vi "Image_Capture.vi"() -> ()   [LabVIEW 2017]
uses:
  <vilib>/vision/NI_Vision_Development_Module.lvlib
panel:
  out "error out":errorcluster
  out "Histogram Report":T1 {"Standard  Variation" format="%.2f"; "Mean Value" format="%.2f"; "Interval Width" format="%.2f"; "Starting Value" format="%.2f"; "Maximal Value" format="%.2f"; "Minimal Value" format="%.2f"}
  in  "Contrast::Value":dbl min=0.0 max=1.0
  in  "Brightness::Value":i64=116 min=0 max=255 step=1
  out "Frame Rate":dbl
  in  "Stop (F)":bool
  out "Image Out":T2(plugin-control)
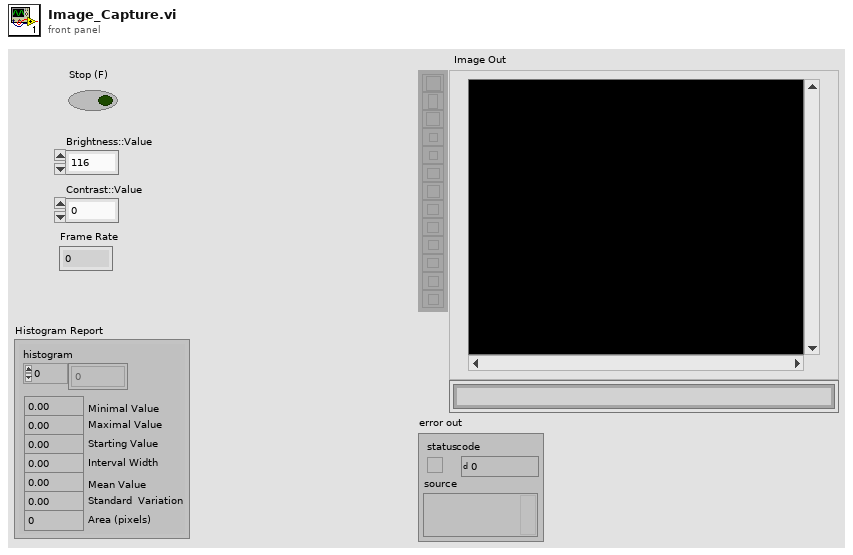
[diagram p1: front panel]
types:
  T1 = cluster{"histogram":u32[], "Minimal Value":sgl, "Maximal Value":sgl, "Starting Value":sgl, "Interval Width":sgl, "Mean Value":sgl, "Standard  Variation":sgl, "Area (pixels)":i32}
  T2 = typedef "IMAQ Image.ctl" = refnum<image>
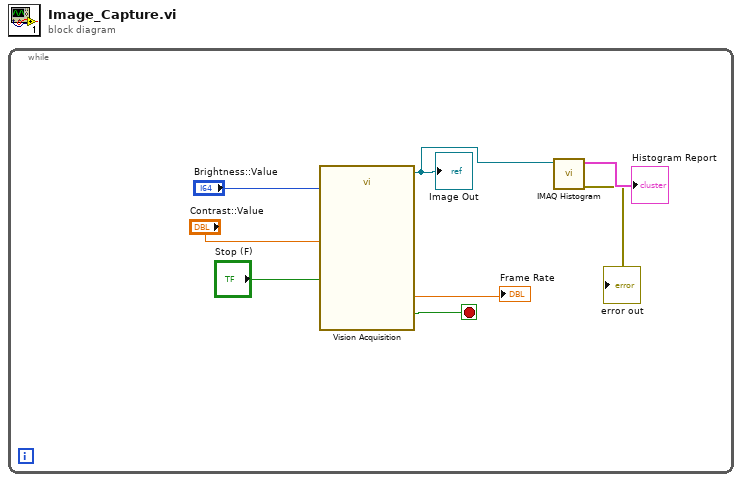
[diagram p0: block diagram]
diagram:
  n1 = while {
    stop <- w7 stop-if-true
    n2 = call "Vision Acquisition"("Brightness::Value"="Brightness::Value", "Contrast::Value"="Contrast::Value", "Stop (F)"="Stop (F)") -> ("Image Out"=w3:T2, "Frame Rate"=→"Frame Rate":dbl, "Stopped"=w7:bool)  [unwired: 21 in, 1 out]
    "Image Out" <- w3
    n3 = call "IMAQ Histogram"("Image"=w3) -> ("error out"=→"error out":errorcluster, "Histogram Report"=→"Histogram Report":T1)  [unwired: 9 in]
  }
